vi "BDSCTRL_Write_Configuration_Settings_File.vi"(0 "configuration file path":path, 1 "BDSCTRL Connection Settings":T9={"Panel IP Address"="10.1.11.247", "Melvitron IP Address"="COM12", "EXA IP Address"="10.1.11.123", "MXG IP Address"="10.1.11.122"}, 2 "Test Setup Settings":T8={"IF Calibration File"=path "IFCalExample.csv", "Beam Lookup Table"=path "BeamLookupTableExample.csv", "Test Environment"=enum."Melvitron", "Panel Mode"=enum."CPRI", "Calibration Mode"=0, "Panel Type"=0, "Band"=0, "Tile"=0, "API Drop"=0} {"API Drop" items=["MAY", "JUNE"]; "Tile" items=["HP-C", "HP-B3"]; "Band" items=["AWS", "PCS-A", "PCS-G"]; "Panel Type" items=["Half", "Full", "Quarter"]; "Calibration Mode" items=["Manual", "SemiAuto", "Auto"]}, 3 "Panel Action Sequence":T6[](array[typedef]) items=["Panel Init", "RF Calibration", "Rotate Beam", "Set RF Frequency", "Initial Calibrations", "Channel Enable", "IF Calibration", "Sense Power", "Measure Temperature", "Set RF Power Level", "Run DMA", "Set RF Bandwidth", "Set CFR", "Set Beam"], 5 "error in \n(no error)":errorcluster, 6 "Channels Cluster":T7={"TX1"=TRUE, "TX2"=TRUE, "TX3"=FALSE, "TX4"=FALSE, "TXx3"=TRUE, "TXx4"=TRUE, "RX1"=FALSE, "RX2"=FALSE, "RX3"=FALSE, "RX4"=FALSE, "RXx3"=FALSE, "RXx4"=FALSE, "Tx"=TRUE, "Rx"=FALSE}, 7 "Set Beam Settings Cluster":T3, 8 "Beam Rotation":string[][](table)=[["1"], ["1"], ["1"], ["1"], ["1"], ["1"], ["2"], ["2"], ["2"], ["2"], ["2"], ["2"]], 9 "DMA Settings Cluster":T2, 10 "Target Devices Cluster":T5={"Target Devices"={"P1 Cluster"={"P1_D1"=TRUE, "P1_D2"=TRUE, "P1_D3"=TRUE, "P1_D4"=TRUE, "P1_D5"=TRUE, "P1_D6"=TRUE, "P1_D7"=TRUE, "P1_D8"=TRUE, "P1_D9"=TRUE, "P1_D10"=TRUE, "P1_D11"=TRUE, "P1_D12"=TRUE, "P1_D13"=TRUE, "P1_D14"=TRUE, "P1_D15"=TRUE, "P1_D16"=TRUE, "P1_D17"=TRUE, "P1_D18"=TRUE, "P1_D19"=TRUE, "P1_D20"=TRUE, "P1_D21"=TRUE, "P1_D22"=TRUE, "P1_D23"=TRUE, "P1_D24"=TRUE}, "P2 Cluster"={"P2_D1"=TRUE, "P2_D2"=TRUE, "P2_D3"=TRUE, "P2_D4"=TRUE, "P2_D5"=TRUE, "P2_D6"=TRUE, "P2_D7"=TRUE, "P2_D8"=TRUE, "P2_D9"=TRUE, "P2_D10"=TRUE, "P2_D11"=TRUE, "P2_D12"=TRUE, "P2_D13"=TRUE, "P2_D14"=TRUE, "P2_D15"=TRUE, "P2_D16"=TRUE, "P2_D17"=TRUE, "P2_D18"=TRUE, "P2_D19"=TRUE, "P2_D20"=TRUE, "P2_D21"=TRUE, "P2_D22"=TRUE, "P2_D23"=TRUE, "P2_D24"=TRUE}}, "Target String"="{1:24,1:24,[],[]}"}, 11 "MB-CFR Settings Cluster":T1, 12 "RF Parameters Settings Cluster":T4={"Tx RF \nFrequency"=2132.5, "RF Bandwidth \n(MHz)"=0, "Tx VGA"=[], "Rx VGA"=[]}) -> (19 "error out":errorcluster)   [LabVIEW 2016]
doc: "Illustrates how to create and write a configuration settings file.\n\nInstructions:\nEnter values in the controls on the front panel then click on the Run Arrow.\nTo read the file, run Read Configuration Settings File.vi located in the file\\config.llb."
uses:
  BDSCTRL_Controls/BDSCTRL_Panel_Action_List.ctl
  <vilib>/Utility/config.llb/Write Key (String).vi
  <vilib>/Utility/config.llb/Write Key (Path).vi
  <vilib>/Utility/config.llb/Write Key (I32).vi
  <vilib>/Utility/config.llb/Write Key (U32).vi
  <vilib>/Utility/config.llb/Write Key (Boolean).vi
  <vilib>/Utility/config.llb/Write Key (Double).vi
  <vilib>/Utility/config.llb/NI_LVConfig.lvlib
panel:
  in  "Instrument Mode Cluster":T10
  out "Array Indexing":string[](array[string])=["A", "B", "C", "D", "E", "F"]
  in  "Test Array":T11(array[cluster])=[{"Test Module"=0, "Select"=TRUE, "Configure\nParameters"=FALSE}, {"Test Module"=0, "Select"=FALSE, "Configure\nParameters"=FALSE}, {"Test Module"=0, "Select"=FALSE, "Configure\nParameters"=FALSE}, {"Test Module"=0, "Select"=FALSE, "Configure\nParameters"=FALSE}, {"Test Module"=0, "Select"=FALSE, "Configure\nParameters"=FALSE}, {"Test Module"=0, "Select"=FALSE, "Configure\nParameters"=FALSE}, {"Test Module"=0, "Select"=FALSE, "Configure\nParameters"=FALSE}, {"Test Module"=0, "Select"=FALSE, "Configure\nParameters"=FALSE}, {"Test Module"=0, "Select"=FALSE, "Configure\nParameters"=FALSE}, {"Test Module"=0, "Select"=FALSE, "Configure\nParameters"=FALSE}, {"Test Module"=0, "Select"=FALSE, "Configure\nParameters"=FALSE}, {"Test Module"=0, "Select"=FALSE, "Configure\nParameters"=FALSE}, {"Test Module"=0, "Select"=FALSE, "Configure\nParameters"=FALSE}, {"Test Module"=0, "Select"=FALSE, "Configure\nParameters"=FALSE}, {"Test Module"=0, "Select"=FALSE, "Configure\nParameters"=FALSE}, {"Test Module"=0, "Select"=FALSE, "Configure\nParameters"=FALSE}, {"Test Module"=0, "Select"=FALSE, "Configure\nParameters"=FALSE}, {"Test Module"=0, "Select"=FALSE, "Configure\nParameters"=FALSE}, {"Test Module"=0, "Select"=FALSE, "Configure\nParameters"=FALSE}, {"Test Module"=0, "Select"=FALSE, "Configure\nParameters"=FALSE}] {"Test Module" items=["::Select_a_module::", "Dynamic_Range", "EVM_FreqErr_OutputPower_GainFlatness", "RSSI"]}
  # "P2"
  # "P1"
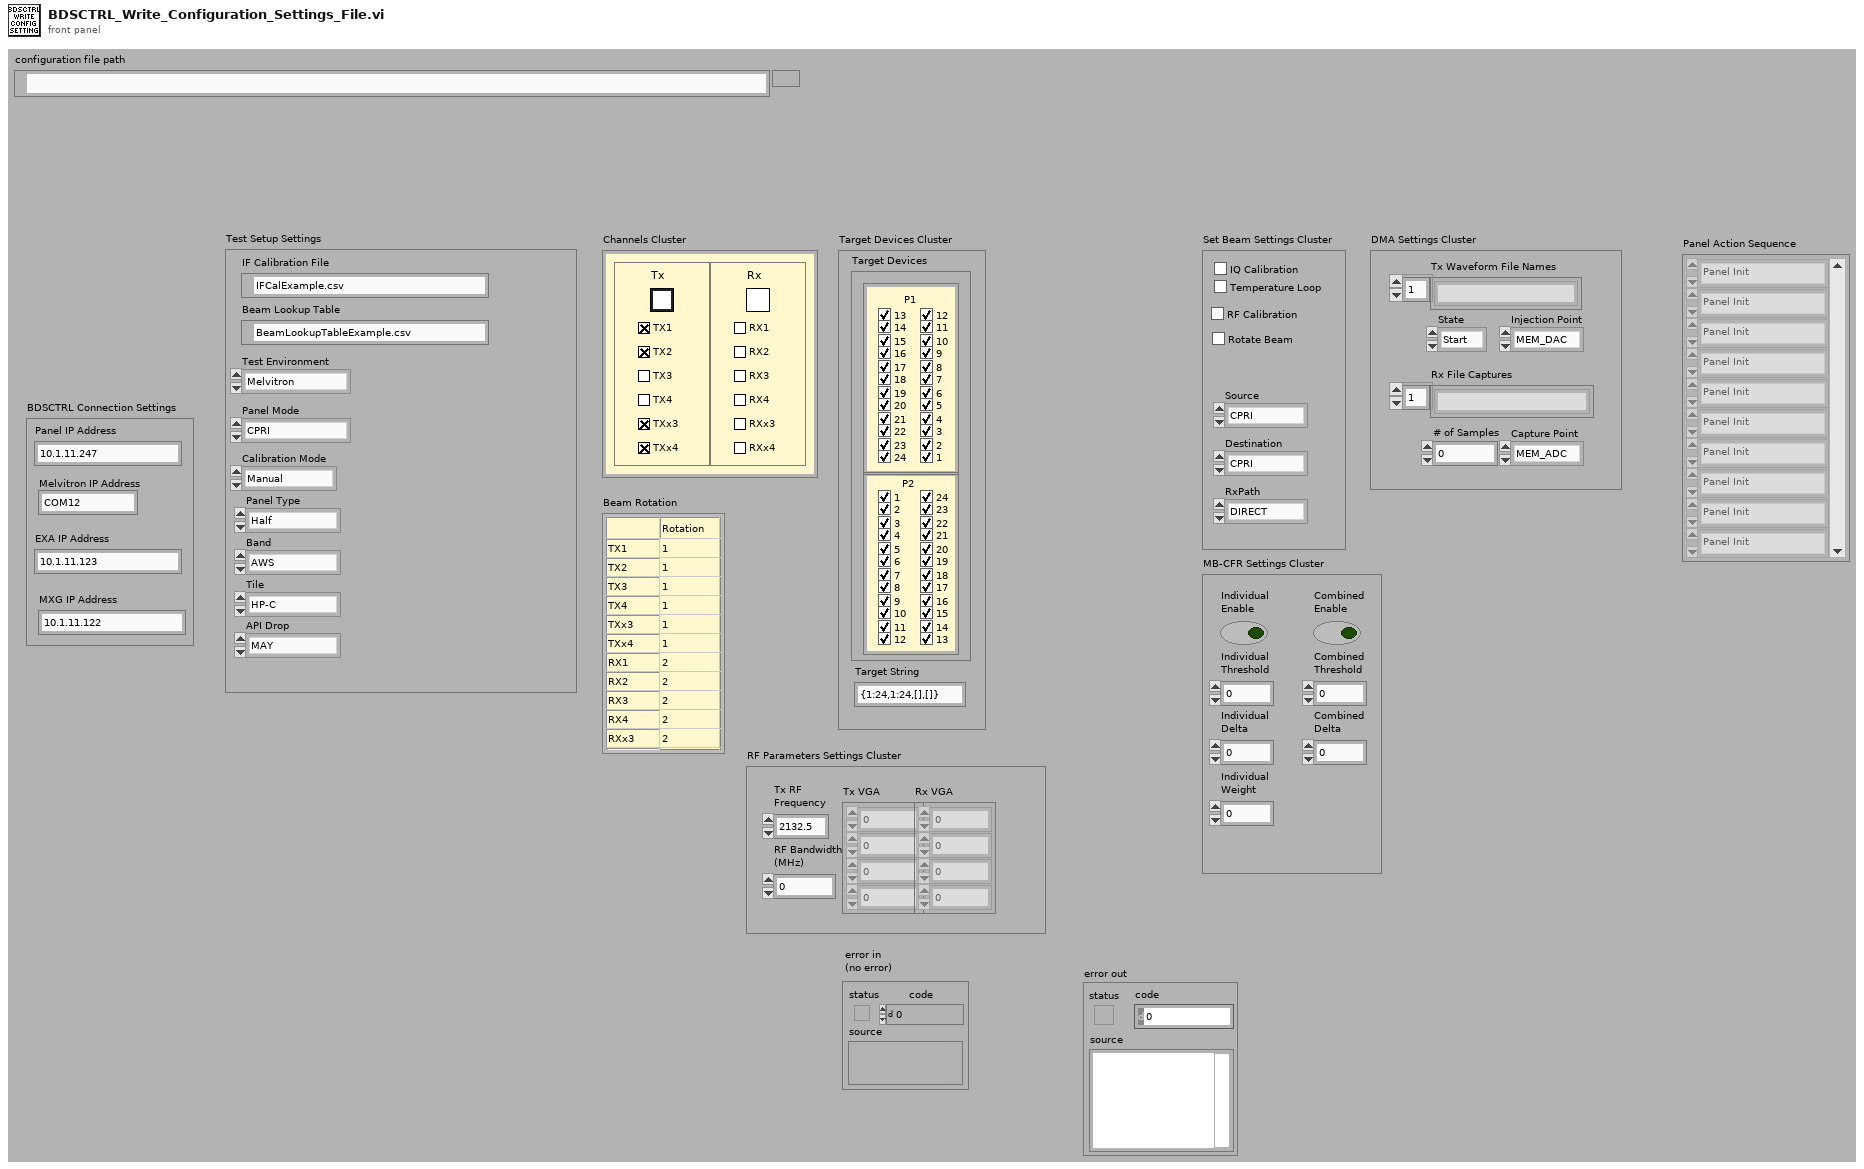
[diagram p1: front panel]
types:
  T1 = cluster{"Individual\nEnable":bool, "Individual\nThreshold":dbl, "Individual\nDelta":dbl, "Individual\nWeight":dbl, "Combined\nEnable":bool, "Combined\nThreshold":dbl, "Combined\nDelta":dbl}
  T2 = cluster{"Tx Waveform File Names":string[], "State":enum16{"Start", "Stop"}, "Injection Point":enum16{"MEM_DAC", "MEM_DUC"}, "Rx File Captures":string[], "# of Samples":i32, "Capture Point":enum16{"MEM_ADC", "MEM_DDC"}}
  T3 = cluster{"IQ Calibration":bool, "Temperature Loop":bool, "RF Calibration":bool, "Rotate Beam":bool, "Source":enum16{"CPRI", "CAL", "MEM_DAC", "MEM_DUC", "EXT"}, "Destination":enum16{"CPRI", "EXT", "MEM_ADC", "MEM_DDC"}, "RxPath":enum16{"DIRECT", "MIXER"}}
  T4 = cluster{"Tx RF \nFrequency":dbl, "RF Bandwidth \n(MHz)":i32, "Tx VGA":i32[], "Rx VGA":i32[]}
  T5 = cluster{"Target Devices":cluster{"P1 Cluster":cluster{"P1_D1":bool, "P1_D2":bool, "P1_D3":bool, "P1_D4":bool, "P1_D5":bool, "P1_D6":bool, "P1_D7":bool, "P1_D8":bool, "P1_D9":bool, "P1_D10":bool, "P1_D11":bool, "P1_D12":bool, "P1_D13":bool, "P1_D14":bool, "P1_D15":bool, "P1_D16":bool, "P1_D17":bool, "P1_D18":bool, "P1_D19":bool, "P1_D20":bool, "P1_D21":bool, "P1_D22":bool, "P1_D23":bool, "P1_D24":bool}, "P2 Cluster":cluster{"P2_D1":bool, "P2_D2":bool, "P2_D3":bool, "P2_D4":bool, "P2_D5":bool, "P2_D6":bool, "P2_D7":bool, "P2_D8":bool, "P2_D9":bool, "P2_D10":bool, "P2_D11":bool, "P2_D12":bool, "P2_D13":bool, "P2_D14":bool, "P2_D15":bool, "P2_D16":bool, "P2_D17":bool, "P2_D18":bool, "P2_D19":bool, "P2_D20":bool, "P2_D21":bool, "P2_D22":bool, "P2_D23":bool, "P2_D24":bool}}, "Target String":string}
  T6 = typedef "BDSCTRL_Panel_Action_List.ctl" = u16
  T7 = cluster{"TX1":bool, "TX2":bool, "TX3":bool, "TX4":bool, "TXx3":bool, "TXx4":bool, "RX1":bool, "RX2":bool, "RX3":bool, "RX4":bool, "RXx3":bool, "RXx4":bool, "Tx":bool, "Rx":bool}
  T8 = cluster{"IF Calibration File":path, "Beam Lookup Table":path, "Test Environment":enum16{"Melvitron", "Spider", "Marinotron"}, "Panel Mode":enum16{"CPRI", "UpDnCnv"}, "Calibration Mode":u16, "Panel Type":u16, "Band":u16, "Tile":u16, "API Drop":u16}
  T9 = cluster{"Panel IP Address":string, "Melvitron IP Address":string, "EXA IP Address":string, "MXG IP Address":string}
  T10 = cluster{"MXA Connection":cluster{"MXA":refnum<visa-resource-name>, "Entry Mode":enum16{"VISA", "IP Address"}}, "MXG1 Connection":cluster{"MXG 1":refnum<visa-resource-name>, "Entry Mode":enum16{"VISA", "IP Address"}}, "MXG2 Connection":cluster{"MXG 2":refnum<visa-resource-name>, "Entry Mode":enum16{"VISA", "IP Address"}}, "MXG3 Connection":cluster{"MXG 3":refnum<visa-resource-name>, "Entry Mode":enum16{"VISA", "IP Address"}}, "ENA Connection":cluster{"ENA":refnum<visa-resource-name>, "Entry Mode":enum16{"VISA", "IP Address"}}}
  T11 = cluster{"Test Module":u16, "Select":bool, "Configure\nParameters":bool}[]
  T12 = cluster{"MXA":refnum<visa-resource-name>, "Entry Mode":enum16{"VISA", "IP Address"}}
  T13 = cluster{"MXG 1":refnum<visa-resource-name>, "Entry Mode":enum16{"VISA", "IP Address"}}
  T14 = cluster{"MXG 2":refnum<visa-resource-name>, "Entry Mode":enum16{"VISA", "IP Address"}}
  T15 = cluster{"MXG 3":refnum<visa-resource-name>, "Entry Mode":enum16{"VISA", "IP Address"}}
  T16 = cluster{"ENA":refnum<visa-resource-name>, "Entry Mode":enum16{"VISA", "IP Address"}}
  T17 = typedef "NI_LVConfig.lvlib/Config Data RefNum.ctl" = refnum<k1>
  T18 = cluster{"P1 Cluster":cluster{"P1_D1":bool, "P1_D2":bool, "P1_D3":bool, "P1_D4":bool, "P1_D5":bool, "P1_D6":bool, "P1_D7":bool, "P1_D8":bool, "P1_D9":bool, "P1_D10":bool, "P1_D11":bool, "P1_D12":bool, "P1_D13":bool, "P1_D14":bool, "P1_D15":bool, "P1_D16":bool, "P1_D17":bool, "P1_D18":bool, "P1_D19":bool, "P1_D20":bool, "P1_D21":bool, "P1_D22":bool, "P1_D23":bool, "P1_D24":bool}, "P2 Cluster":cluster{"P2_D1":bool, "P2_D2":bool, "P2_D3":bool, "P2_D4":bool, "P2_D5":bool, "P2_D6":bool, "P2_D7":bool, "P2_D8":bool, "P2_D9":bool, "P2_D10":bool, "P2_D11":bool, "P2_D12":bool, "P2_D13":bool, "P2_D14":bool, "P2_D15":bool, "P2_D16":bool, "P2_D17":bool, "P2_D18":bool, "P2_D19":bool, "P2_D20":bool, "P2_D21":bool, "P2_D22":bool, "P2_D23":bool, "P2_D24":bool}}
  T19 = cluster{"P2_D1":bool, "P2_D2":bool, "P2_D3":bool, "P2_D4":bool, "P2_D5":bool, "P2_D6":bool, "P2_D7":bool, "P2_D8":bool, "P2_D9":bool, "P2_D10":bool, "P2_D11":bool, "P2_D12":bool, "P2_D13":bool, "P2_D14":bool, "P2_D15":bool, "P2_D16":bool, "P2_D17":bool, "P2_D18":bool, "P2_D19":bool, "P2_D20":bool, "P2_D21":bool, "P2_D22":bool, "P2_D23":bool, "P2_D24":bool}[]
  T20 = cluster{"P2_D1":bool, "P2_D2":bool, "P2_D3":bool, "P2_D4":bool, "P2_D5":bool, "P2_D6":bool, "P2_D7":bool, "P2_D8":bool, "P2_D9":bool, "P2_D10":bool, "P2_D11":bool, "P2_D12":bool, "P2_D13":bool, "P2_D14":bool, "P2_D15":bool, "P2_D16":bool, "P2_D17":bool, "P2_D18":bool, "P2_D19":bool, "P2_D20":bool, "P2_D21":bool, "P2_D22":bool, "P2_D23":bool, "P2_D24":bool}
  T21 = enum16{"CPRI", "CAL", "MEM_DAC", "MEM_DUC", "EXT"}
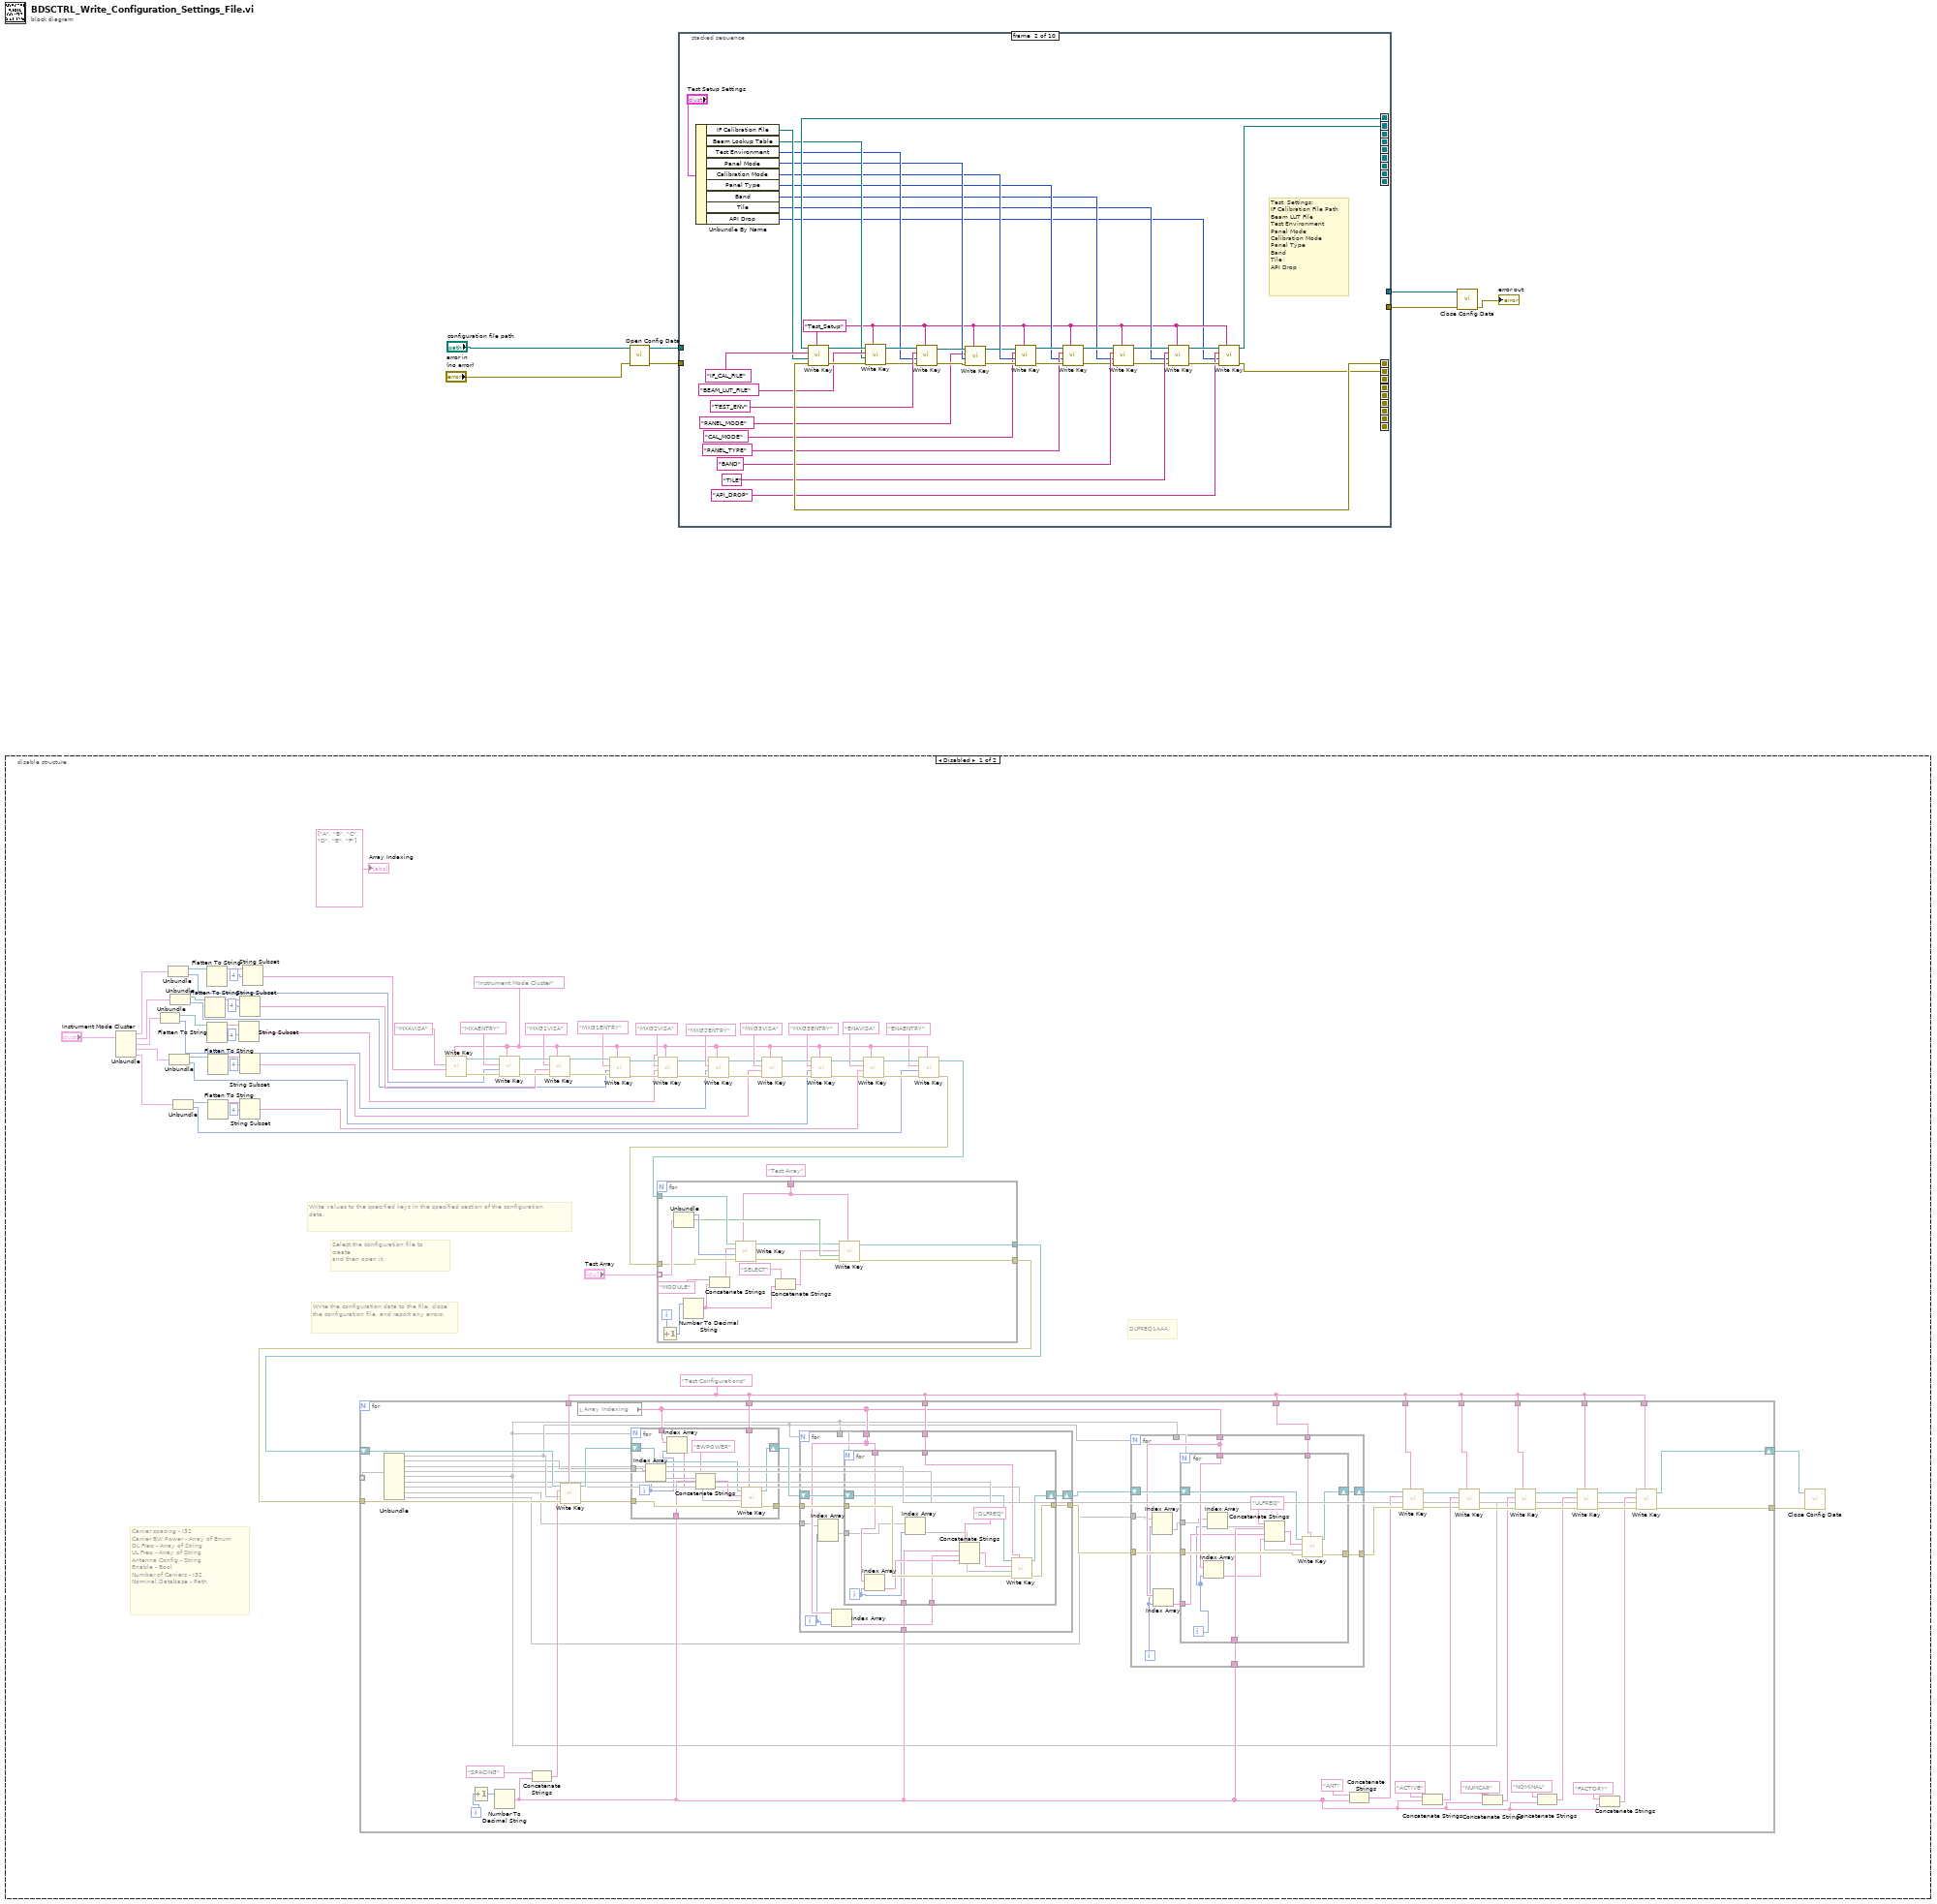
[diagram p0: block diagram]
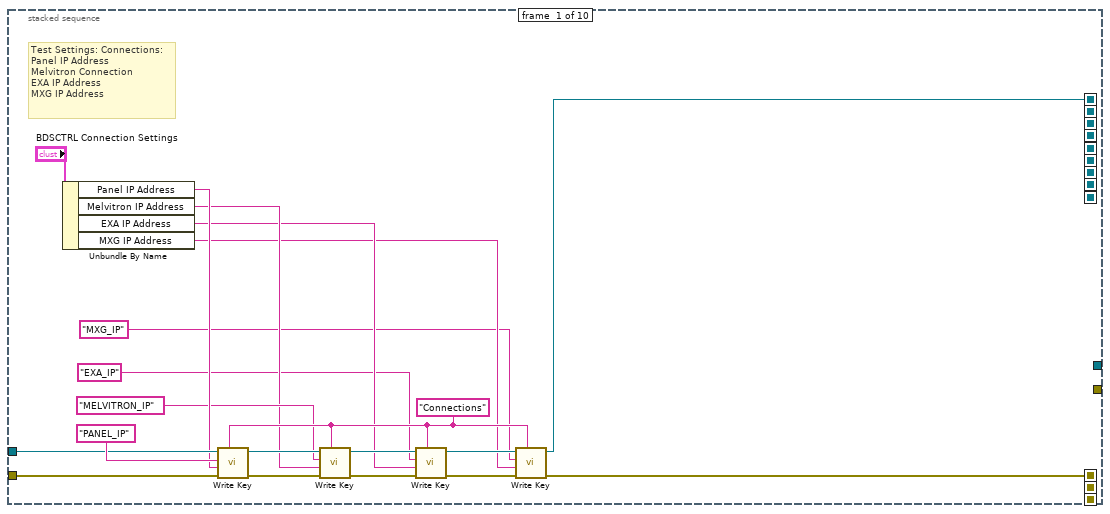
[diagram p3: hidden frame]
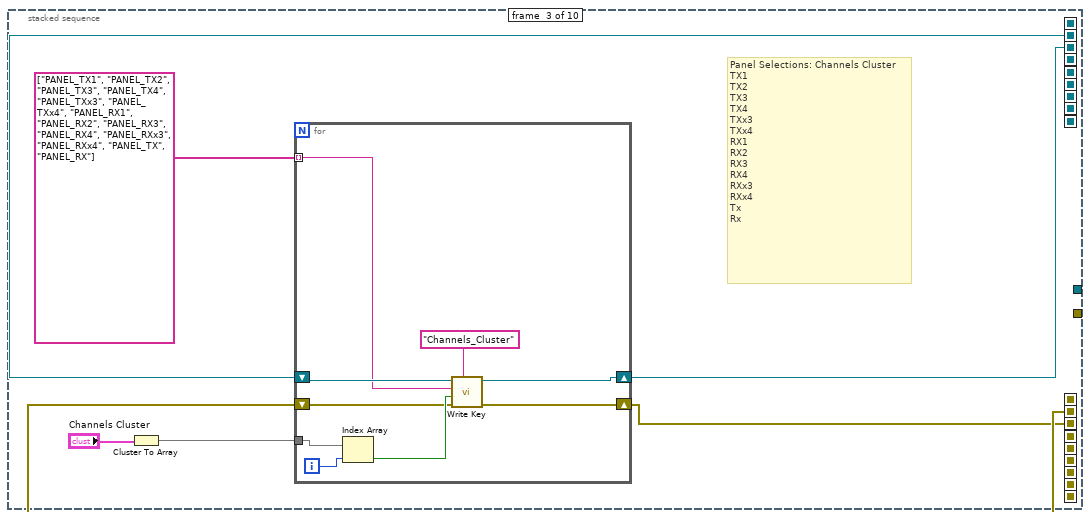
[diagram p4: hidden frame]
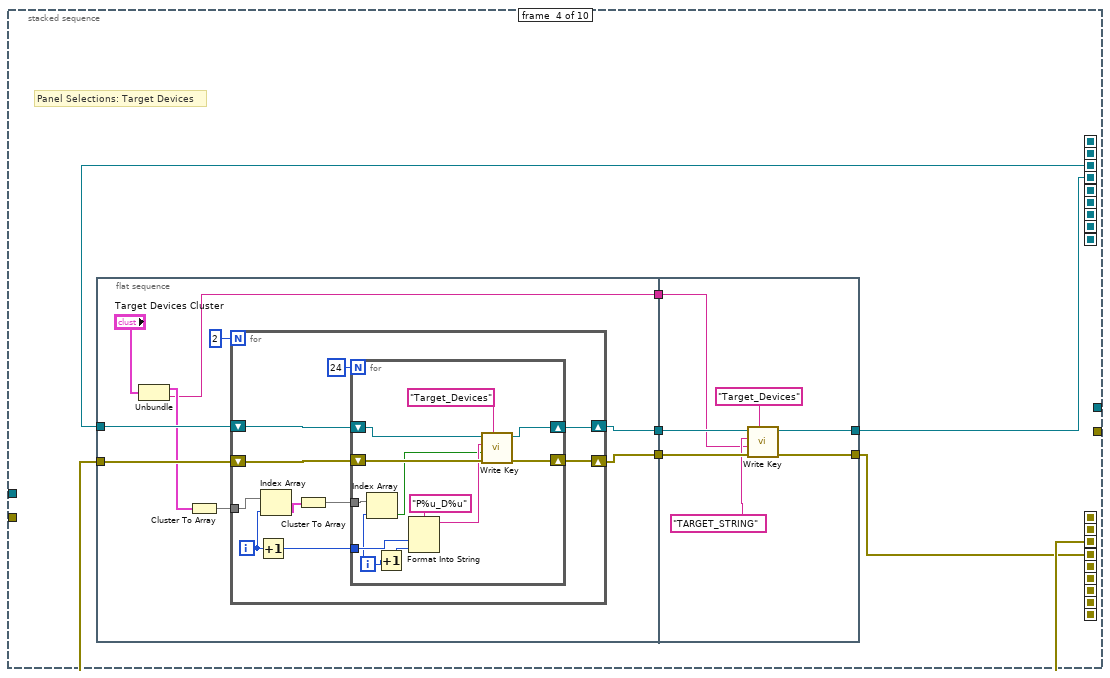
[diagram p5: hidden frame]
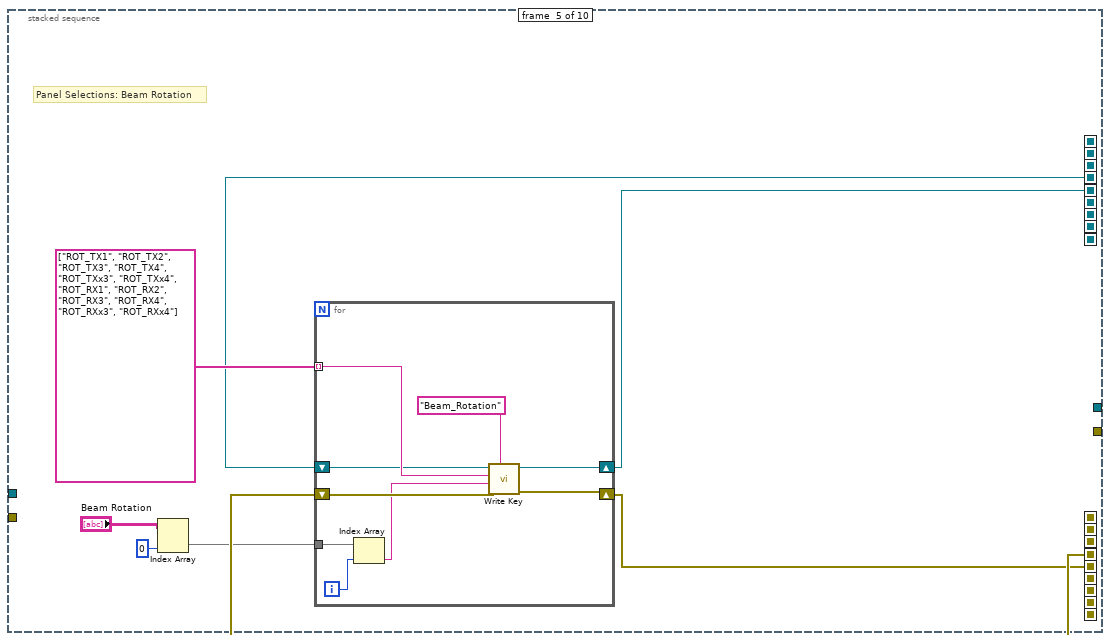
[diagram p6: hidden frame]
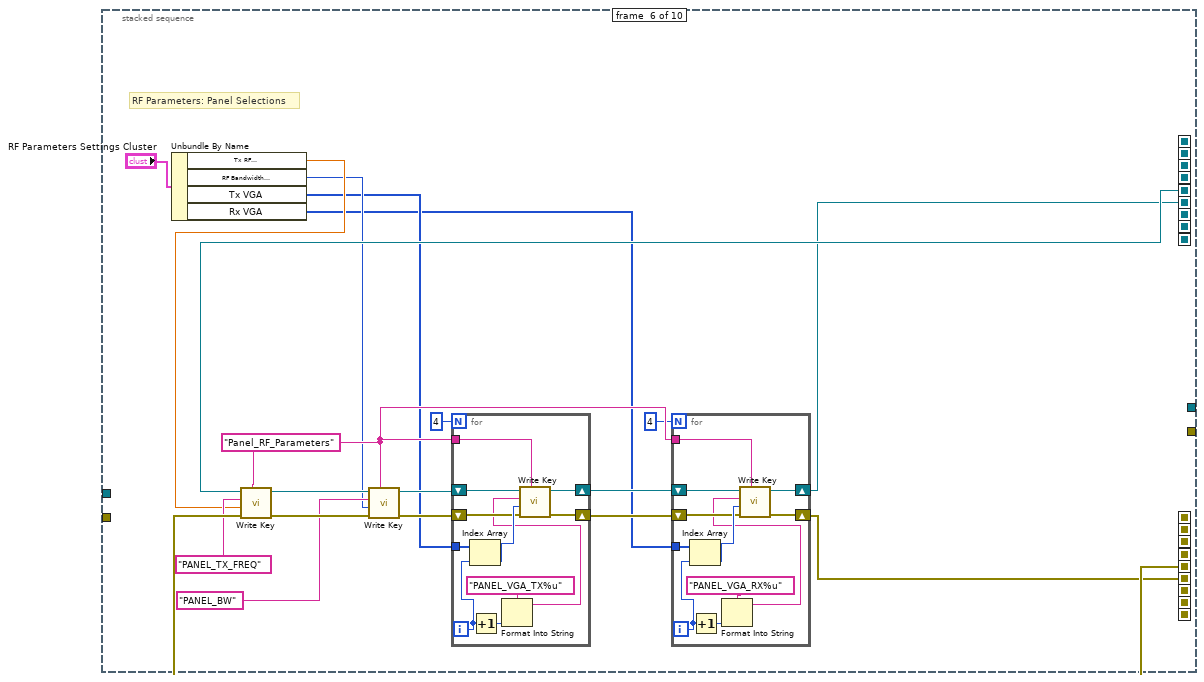
[diagram p7: hidden frame]
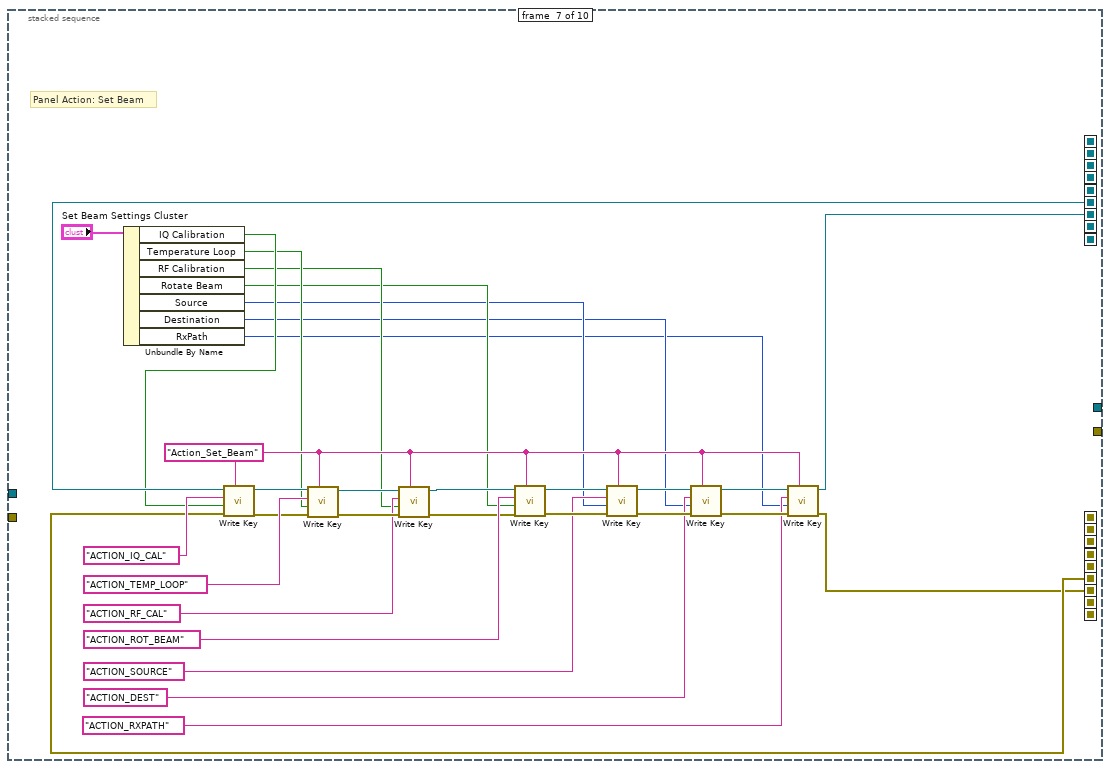
[diagram p8: hidden frame]
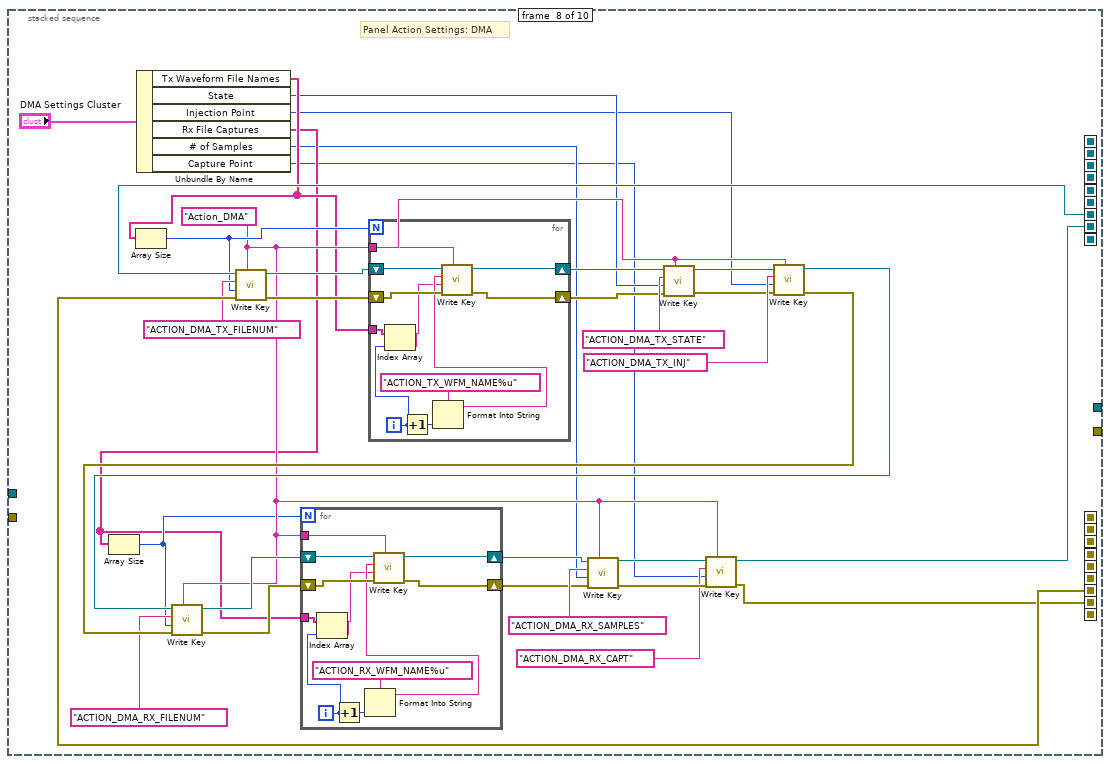
[diagram p9: hidden frame]
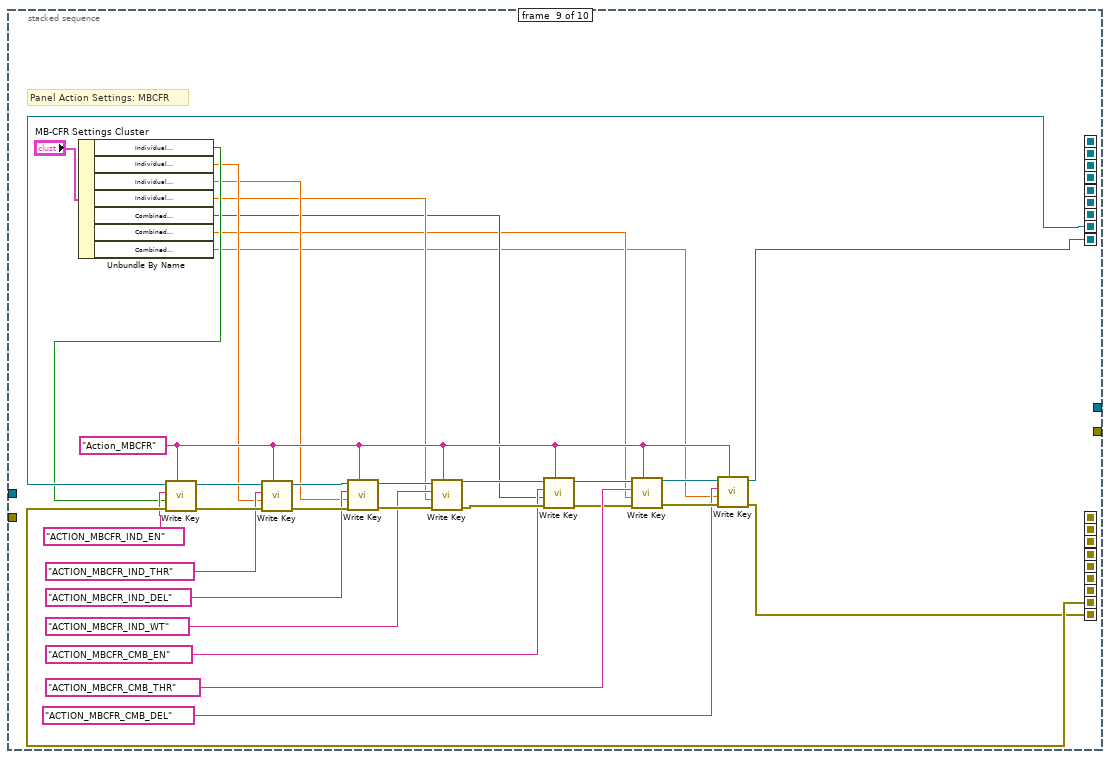
[diagram p10: hidden frame]
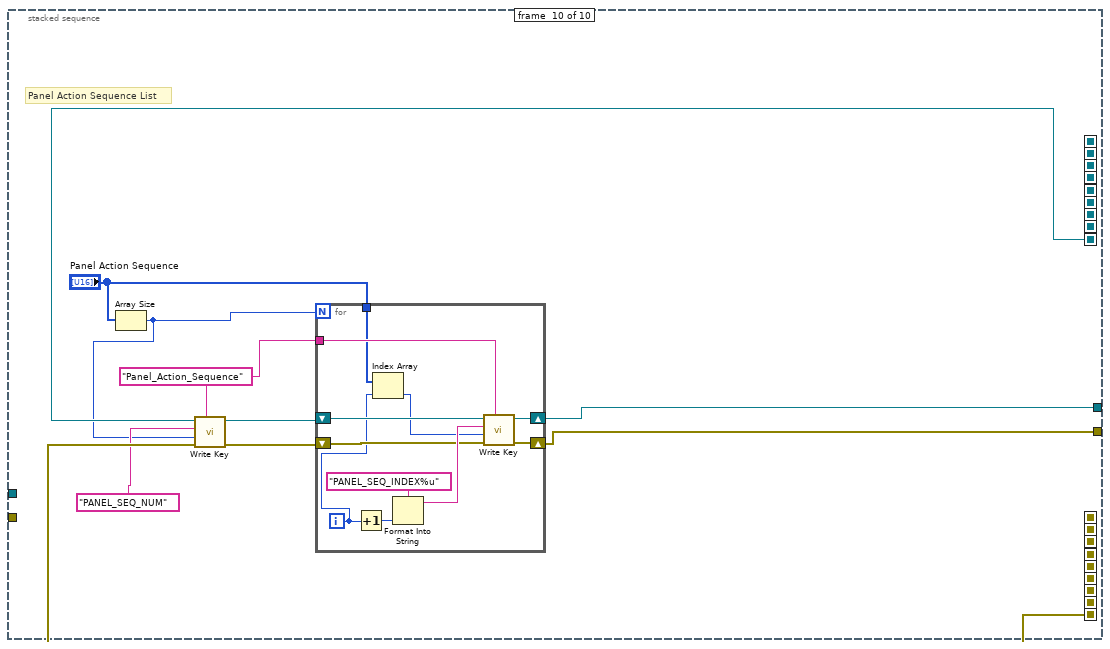
[diagram p11: hidden frame]
diagram:
  n1 = disable-structure shown="Disabled" {
    frame Disabled {
      w12 = "Instrument Mode Cluster" ("section")
      w72 = "Test Configurations" ("section")
      # "DLFREQ1AAA"
      # "Carrier spacing - I32\nCarrier BW Power - Array of Enum\nDL Freq - Array of String\nUL Freq - Array of String\nAntenna Config - String\nEnable - Bool\nNumber of Carriers - I32\nNominal Database - Path"
      # "Write the configuration data to the file, close the configuration file, and report any errors."
      # "Write values to the specified keys in the specified section of the configuration data."
      # "Select the configuration file to create\nand then open it."
      n2 = Unbundle("Instrument Mode Cluster") -> ("MXA Connection"=w70:T12, "MXG1 Connection"=w69:T13, "MXG2 Connection"=w68:T14, "MXG3 Connection"=w67:T15, "ENA Connection"=w66:T16)
      n3 = Unbundle(w68) -> ("MXG 2"=w55:refnum<visa-resource-name>, "Entry Mode"=w26:enum16{"VISA", "IP Address"})
      n4 = Unbundle(w70) -> ("MXA"=w61:refnum<visa-resource-name>, "Entry Mode"=w43:enum16{"VISA", "IP Address"})
      n5 = Unbundle(w67) -> ("MXG 3"=w53:refnum<visa-resource-name>, "Entry Mode"=w20:enum16{"VISA", "IP Address"})
      n6 = Unbundle(w69) -> ("MXG 1"=w58:refnum<visa-resource-name>, "Entry Mode"=w31:enum16{"VISA", "IP Address"})
      n7 = Unbundle(w66) -> ("ENA"=w51:refnum<visa-resource-name>, "Entry Mode"=w10:enum16{"VISA", "IP Address"})
      n8 = Flatten To String(anything=w58) -> (data string=w60:string)  [unwired: 3 in, 2 out]
      n9 = Flatten To String(anything=w61) -> (data string=w62:string)  [unwired: 3 in, 2 out]
      n10 = Flatten To String(anything=w55) -> (data string=w56:string)  [unwired: 3 in, 2 out]
      n11 = Flatten To String(anything=w53) -> (data string=w52:string)  [unwired: 3 in, 2 out]
      n12 = Flatten To String(anything=w51) -> (data string=w49:string)  [unwired: 3 in, 2 out]
      n13 = String Subset(string=w56, offset (0)=4) -> (substring=w32:string)  [unwired: 1 in]
      n14 = String Subset(string=w52, offset (0)=4) -> (substring=w23:string)  [unwired: 1 in]
      n15 = String Subset(string=w60, offset (0)=4) -> (substring=w39:string)  [unwired: 1 in]
      n16 = String Subset(string=w49, offset (0)=4) -> (substring=w17:string)  [unwired: 1 in]
      n17 = String Subset(string=w62, offset (0)=4) -> (substring=w47:string)  [unwired: 1 in]
      n18 = call-poly <vilib>:"Write Key.vi"("section"=w12, "value"=w47, "key"="MXAVISA") -> ("error out"=w45:errorcluster, "refnum out"=w46:T17, "error in (no error)"=w64:errorcluster, "refnum"=w65:T17)  [unwired: 4 in, 1 out]
      n19 = call-poly <vilib>:"Write Key.vi"("section"=w12, "error in (no error)"=w45, "value"=w43, "key"="MXAENTRY", "refnum"=w46) -> ("error out"=w41:errorcluster, "refnum out"=w42:T17)  [unwired: 4 in, 1 out]
      n20 = call-poly <vilib>:"Write Key.vi"("section"=w12, "error in (no error)"=w41, "value"=w39, "key"="MXG1VISA", "refnum"=w42) -> ("error out"=w38:errorcluster, "refnum out"=w37:T17)  [unwired: 4 in, 1 out]
      n21 = call-poly <vilib>:"Write Key.vi"("section"=w12, "error in (no error)"=w38, "value"=w31, "key"="MXG1ENTRY", "refnum"=w37) -> ("error out"=w34:errorcluster, "refnum out"=w35:T17)  [unwired: 4 in, 1 out]
      n22 = call-poly <vilib>:"Write Key.vi"("section"=w12, "error in (no error)"=w34, "value"=w32, "key"="MXG2VISA", "refnum"=w35) -> ("error out"=w30:errorcluster, "refnum out"=w27:T17)  [unwired: 4 in, 1 out]
      n23 = call-poly <vilib>:"Write Key.vi"("section"=w12, "error in (no error)"=w30, "value"=w26, "key"="MXG2ENTRY", "refnum"=w27) -> ("error out"=w29:errorcluster, "refnum out"=w24:T17)  [unwired: 4 in, 1 out]
      n24 = call-poly <vilib>:"Write Key.vi"("section"=w12, "error in (no error)"=w29, "value"=w23, "key"="MXG3VISA", "refnum"=w24) -> ("error out"=w22:errorcluster, "refnum out"=w21:T17)  [unwired: 4 in, 1 out]
      n25 = call-poly <vilib>:"Write Key.vi"("section"=w12, "error in (no error)"=w22, "value"=w20, "key"="MXG3ENTRY", "refnum"=w21) -> ("error out"=w16:errorcluster, "refnum out"=w15:T17)  [unwired: 4 in, 1 out]
      n26 = call-poly <vilib>:"Write Key.vi"("section"=w12, "error in (no error)"=w16, "value"=w17, "key"="ENAVISA", "refnum"=w15) -> ("error out"=w14:errorcluster, "refnum out"=w13:T17)  [unwired: 4 in, 1 out]
      n27 = call-poly <vilib>:"Write Key.vi"("section"=w12, "error in (no error)"=w14, "value"=w10, "key"="ENAENTRY", "refnum"=w13) -> ("error out"=w8:errorcluster, "refnum out"=w9:T17)  [unwired: 4 in, 1 out]
      n28 = for {
        tunnel: "Test Array" ("section") -> [w205]
        tunnel: [w202] -> w75
        tunnel: [w203] -> w77
        tunnel: "Test Array" -> [w215] mode=indexing
        tunnel: w8 -> [w214]
        tunnel: w9 -> [w211]
        i -> [w218]
        n29 = Increment(x=w218) -> (x+1=w216:i32)
        n30 = Unbundle(w215) -> ("Test Module"=w213:u16, "Select"=w208:bool)  [unwired: 1 out]
        n31 = Number To Decimal String(number=w216) -> (decimal integer string=w209:string)  [unwired: 1 in]
        n32 = Concatenate Strings("MODULE", w209) -> (w212:string)
        n33 = call-poly <vilib>:"Write Key.vi"("section"=w205, "error in (no error)"=w214, "value"=w213, "key"=w212, "refnum"=w211) -> ("error out"=w204:errorcluster, "refnum out"=w207:T17)  [unwired: 4 in, 1 out]
        n34 = Concatenate Strings("SELECT", w209) -> (w206:string)
        n35 = call-poly <vilib>:"Write Key.vi"("section"=w205, "error in (no error)"=w204, "value"=w208, "key"=w206, "refnum"=w207) -> ("error out"=w203:errorcluster, "refnum out"=w202:T17)  [unwired: 4 in, 1 out]
      }
      n36 = for {
        tunnel: [w136] -> w78 mode=indexing
        tunnel: w77 -> [w133]
        tunnel: w72 -> [w132]
        tunnel: w72 -> [w127]
        tunnel: w72 -> [w125]
        tunnel: w72 -> [w122]
        tunnel: w72 -> [w118]
        tunnel: w72 -> [w111]
        tunnel: w72 -> [w108]
        shift-right: [w91] -> w73
        shift-left: w75 -> [w105]
        tunnel: [w90] -> w74
        tunnel: w72 -> [w101]
        tunnel: w72 -> [w99]
        i -> [w134]
        n37 = Unbundle(w136) -> (w87, w130, w86, w85, w84, w83, w82, w89, w88)
        n38 = Increment(x=w134) -> (x+1=w135:i32)
        n39 = Number To Decimal String(number=w135) -> (decimal integer string=w94:string)  [unwired: 1 in]
        n40 = Concatenate Strings("SPACING", w94) -> (w121:string)
        n41 = call-poly <vilib>:"Write Key.vi"("section"=w132, "error in (no error)"=w133, "value"=w87, "key"=w121, "refnum"=w105) -> ("error out"=w128:errorcluster, "refnum out"=w129:T17)  [unwired: 4 in, 1 out]
        n42 = local read "Array Indexing"() -> (w124:string[])
        n43 = for {
          N: w84 -> [_]
          tunnel: w130 -> [w201]
          shift-right: [w195] -> w104
          shift-left: w129 -> [w196]
          tunnel: w128 -> [w200]
          tunnel: w124 -> [w191]
          tunnel: w94 -> [w199]
          tunnel: w127 -> [w194]
          tunnel: [w192] -> w126
          i -> [w190]
          n44 = Index Array(array=w201, index=w190) -> (element=w193)
          n45 = Index Array(array=w191, index=w190) -> (element=w189:string)
          n46 = Concatenate Strings("BWPOWER", w199, w189) -> (w197:string)
          n47 = call-poly <vilib>:"Write Key.vi"("section"=w194, "error in (no error)"=w200, "value"=w193, "key"=w197, "refnum"=w196) -> ("error out"=w192:errorcluster, "refnum out"=w195:T17)  [unwired: 4 in, 1 out]
        }
        n48 = for {
          N: w87 -> [_]
          tunnel: w126 -> [w174]
          tunnel: w89 -> [w166]
          tunnel: w125 -> [w173]
          tunnel: w124 -> [w168]
          tunnel: [w171] -> w123
          tunnel: w94 -> [w170]
          shift-right: [w172] -> w103
          shift-left: w104 -> [w169]
          tunnel: w84 -> [w165]
          i -> [w164]
          n49 = Index Array(array=w166, index (row)=w164) -> (element=w163)  [unwired: 1 in]
          n50 = Index Array(array=w168, index=w164) -> (element=w167:string)
          n51 = for {
            N: w165 -> [_]
            tunnel: w174 -> [w188]
            tunnel: w173 -> [w187]
            tunnel: w168 -> [w182]
            tunnel: [w185] -> w171
            tunnel: w170 -> [w184]
            shift-right: [w186] -> w172
            shift-left: w169 -> [w183]
            tunnel: w167 -> [w178]
            tunnel: w163 -> [w177]
            i -> [w176]
            n52 = Index Array(array=w182, index=w176) -> (element=w179:string)
            n53 = Index Array(array=w177, index=w176) -> (element=w175)
            n54 = Concatenate Strings("DLFREQ", w184, w178, w179) -> (w180:string)
            n55 = call-poly <vilib>:"Write Key.vi"("section"=w187, "error in (no error)"=w188, "value"=w175, "key"=w180, "refnum"=w183) -> ("error out"=w185:errorcluster, "refnum out"=w186:T17)  [unwired: 4 in, 1 out]
          }
        }
        n56 = for {
          N: w87 -> [_]
          tunnel: w124 -> [w142]
          tunnel: w123 -> [w148]
          tunnel: w122 -> [w147]
          tunnel: w88 -> [w140]
          tunnel: [w146] -> w120
          tunnel: w94 -> [w144]
          shift-right: [w145] -> w119
          shift-left: w103 -> [w143]
          tunnel: w84 -> [w137]
          i -> [w139]
          n57 = Index Array(array=w140, index (row)=w139) -> (element=w138)  [unwired: 1 in]
          n58 = Index Array(array=w142, index=w139) -> (element=w141:string)
          n59 = for {
            N: w137 -> [_]
            tunnel: w142 -> [w156]
            tunnel: w148 -> [w162]
            tunnel: w147 -> [w161]
            tunnel: [w160] -> w146
            tunnel: w144 -> [w158]
            shift-right: [w159] -> w145
            shift-left: w143 -> [w157]
            tunnel: w141 -> [w153]
            tunnel: w138 -> [w151]
            i -> [w150]
            n60 = Index Array(array=w156, index=w150) -> (element=w152:string)
            n61 = Index Array(array=w151, index=w150) -> (element=w149)
            n62 = Concatenate Strings("ULFREQ", w158, w153, w152) -> (w154:string)
            n63 = call-poly <vilib>:"Write Key.vi"("section"=w161, "error in (no error)"=w162, "value"=w149, "key"=w154, "refnum"=w157) -> ("error out"=w160:errorcluster, "refnum out"=w159:T17)  [unwired: 4 in, 1 out]
          }
        }
        n64 = Concatenate Strings("ANT", w94) -> (w116:string)
        n65 = call-poly <vilib>:"Write Key.vi"("section"=w118, "error in (no error)"=w120, "value"=w86, "key"=w116, "refnum"=w119) -> ("error out"=w112:errorcluster, "refnum out"=w113:T17)  [unwired: 4 in, 1 out]
        n66 = Concatenate Strings("ACTIVE", w94) -> (w114:string)
        n67 = call-poly <vilib>:"Write Key.vi"("section"=w111, "error in (no error)"=w112, "value"=w85, "key"=w114, "refnum"=w113) -> ("error out"=w110:errorcluster, "refnum out"=w109:T17)  [unwired: 4 in, 1 out]
        n68 = Concatenate Strings("NUMCAR", w94) -> (w106:string)
        n69 = call-poly <vilib>:"Write Key.vi"("section"=w108, "error in (no error)"=w110, "value"=w84, "key"=w106, "refnum"=w109) -> ("error out"=w102:errorcluster, "refnum out"=w96:T17)  [unwired: 4 in, 1 out]
        n70 = Concatenate Strings("NOMINAL", w94) -> (w97:string)
        n71 = call-poly <vilib>:"Write Key.vi"("section"=w101, "error in (no error)"=w102, "value"=w83, "key"=w97, "refnum"=w96) -> ("error out"=w100:errorcluster, "refnum out"=w92:T17)  [unwired: 4 in, 1 out]
        n72 = Concatenate Strings("FACTORY", w94) -> (w93:string)
        n73 = call-poly <vilib>:"Write Key.vi"("section"=w99, "error in (no error)"=w100, "value"=w82, "key"=w93, "refnum"=w92) -> ("error out"=w90:errorcluster, "refnum out"=w91:T17)  [unwired: 4 in, 1 out]
      }
      n74 = call <vilib>:"Close Config Data.vi"("error in (no error)"=w74, "refnum"=w73) -> ("error out"=w81:errorcluster)  [unwired: 1 in, 8 out]
      "Array Indexing" <- string[] ["A", "B", "C", "D", "E", "F"]
    }
    frame Enabled {
    }
  }
  n75 = call <vilib>:"Open Config Data.vi"("error in (no error)"="error in \n(no error)", "configuration file path"="configuration file path") -> ("error out"=w4:errorcluster, "refnum"=w5:T17)  [unwired: 1 in, 7 out]
  n76 = stacked-sequence {
    seq-local: [w220 _ _ _ _ _ _ _ _ _] -> [_ w276 _ _ _ _ _ _ _ _]
    seq-local: [w219 _ _ _ _ _ _ _ _ _] -> [_ w277 _ _ _ _ _ _ _ _]
    seq-local: [_ w240 _ _ _ _ _ _ _ _] -> [_ _ w281 _ _ _ _ _ _ _]
    seq-local: [_ w239 _ _ _ _ _ _ _ _] -> [_ _ w282 _ _ _ _ _ _ _]
    seq-local: [_ _ w279 _ _ _ _ _ _ _] -> [_ _ _ w301 _ _ _ _ _ _]
    seq-local: [_ _ w280 _ _ _ _ _ _ _] -> [_ _ _ w300 _ _ _ _ _ _]
    seq-local: [_ _ _ w297 _ _ _ _ _ _] -> [_ _ _ _ w345 _ _ _ _ _]
    seq-local: [_ _ _ w296 _ _ _ _ _ _] -> [_ _ _ _ w346 _ _ _ _ _]
    seq-local: [_ _ _ _ w341 _ _ _ _ _] -> [_ _ _ _ _ w374 _ _ _ _]
    seq-local: [_ _ _ _ w340 _ _ _ _ _] -> [_ _ _ _ _ w376 _ _ _ _]
    seq-local: [_ _ _ _ _ w363 _ _ _ _] -> [_ _ _ _ _ _ w430 _ _ _]
    seq-local: [_ _ _ _ _ w362 _ _ _ _] -> [_ _ _ _ _ _ w428 _ _ _]
    seq-local: [_ _ _ _ _ _ w407 _ _ _] -> [_ _ _ _ _ _ _ w463 _ _]
    seq-local: [_ _ _ _ _ _ w408 _ _ _] -> [_ _ _ _ _ _ _ w464 _ _]
    seq-local: [_ _ _ _ _ _ _ w440 _ _] -> [_ _ _ _ _ _ _ _ w517 _]
    seq-local: [_ _ _ _ _ _ _ w439 _ _] -> [_ _ _ _ _ _ _ _ w518 _]
    seq-local: [_ _ _ _ _ _ _ _ w496 _] -> [_ _ _ _ _ _ _ _ _ w528]
    seq-local: [_ _ _ _ _ _ _ _ w495 _] -> [_ _ _ _ _ _ _ _ _ w527]
    tunnel: w5 -> [w231 _ _ _ _ _ _ _ _ _]
    tunnel: w4 -> [w230 _ _ _ _ _ _ _ _ _]
    tunnel: [_ _ _ _ _ _ _ _ _ w521] -> w2
    tunnel: [_ _ _ _ _ _ _ _ _ w520] -> w1
    frame #0 {
      w229 = "Connections" ("section")
      # "Test Settings: Connections:\nPanel IP Address\nMelvitron Connection\nEXA IP Address\nMXG IP Address"
      n77 = Unbundle By Name("BDSCTRL Connection Settings") -> ("Panel IP Address"=w227:string, "Melvitron IP Address"=w225:string, "EXA IP Address"=w224:string, "MXG IP Address"=w222:string)
      n78 = call-poly <vilib>:"Write Key.vi"("section"=w229, "error in (no error)"=w230, "value"=w227, "key"="PANEL_IP", "refnum"=w231) -> ("error out"=w235:errorcluster, "refnum out"=w238:T17)  [unwired: 4 in, 1 out]
      n79 = call-poly <vilib>:"Write Key.vi"("section"=w229, "error in (no error)"=w235, "value"=w225, "key"="MELVITRON_IP", "refnum"=w238) -> ("error out"=w234:errorcluster, "refnum out"=w237:T17)  [unwired: 4 in, 1 out]
      n80 = call-poly <vilib>:"Write Key.vi"("section"=w229, "error in (no error)"=w234, "value"=w224, "key"="EXA_IP", "refnum"=w237) -> ("error out"=w233:errorcluster, "refnum out"=w236:T17)  [unwired: 1 in, 4 out]
      n81 = call-poly <vilib>:"Write Key.vi"("section"=w229, "error in (no error)"=w233, "value"=w222, "key"="MXG_IP", "refnum"=w236) -> ("error out"=w219:errorcluster, "refnum out"=w220:T17)  [unwired: 1 in, 4 out]
    }
    frame #1 {
      w243 = "Test_Setup" ("section")
      # "Test  Settings:\nIF Calibration File Path\nBeam LUT File\nTest Environment\nPanel Mode\nCalibration Mode\nPanel Type\nBand\nTile\nAPI Drop"
      n82 = Unbundle By Name("Test Setup Settings") -> ("IF Calibration File"=w273:path, "Beam Lookup Table"=w270:path, "Test Environment"=w266:enum16{"Melvitron", "Spider", "Marinotron"}, "Panel Mode"=w263:enum16{"CPRI", "UpDnCnv"}, "Calibration Mode"=w261:u16, "Panel Type"=w254:u16, "Band"=w251:u16, "Tile"=w246:u16, "API Drop"=w241:u16)
      n83 = call-poly <vilib>:"Write Key.vi"("section"=w243, "error in (no error)"=w277, "value"=w273, "key"="IF_CAL_FILE", "refnum"=w276) -> ("error out"=w272:errorcluster, "refnum out"=w274:T17)  [unwired: 4 in, 1 out]
      n84 = call-poly <vilib>:"Write Key.vi"("section"=w243, "error in (no error)"=w272, "value"=w270, "key"="BEAM_LUT_FILE", "refnum"=w274) -> ("error out"=w268:errorcluster, "refnum out"=w267:T17)  [unwired: 4 in, 1 out]
      n85 = call-poly <vilib>:"Write Key.vi"("section"=w243, "error in (no error)"=w268, "value"=w266, "key"="TEST_ENV", "refnum"=w267) -> ("error out"=w265:errorcluster, "refnum out"=w264:T17)  [unwired: 4 in, 1 out]
      n86 = call-poly <vilib>:"Write Key.vi"("section"=w243, "error in (no error)"=w265, "value"=w263, "key"="PANEL_MODE", "refnum"=w264) -> ("error out"=w259:errorcluster, "refnum out"=w260:T17)  [unwired: 4 in, 1 out]
      n87 = call-poly <vilib>:"Write Key.vi"("section"=w243, "error in (no error)"=w259, "value"=w261, "key"="CAL_MODE", "refnum"=w260) -> ("error out"=w257:errorcluster, "refnum out"=w256:T17)  [unwired: 4 in, 1 out]
      n88 = call-poly <vilib>:"Write Key.vi"("section"=w243, "error in (no error)"=w257, "value"=w254, "key"="PANEL_TYPE", "refnum"=w256) -> ("error out"=w250:errorcluster, "refnum out"=w253:T17)  [unwired: 4 in, 1 out]
      n89 = call-poly <vilib>:"Write Key.vi"("section"=w243, "error in (no error)"=w250, "value"=w251, "key"="BAND", "refnum"=w253) -> ("error out"=w247:errorcluster, "refnum out"=w249:T17)  [unwired: 4 in, 1 out]
      n90 = call-poly <vilib>:"Write Key.vi"("section"=w243, "error in (no error)"=w247, "value"=w246, "key"="TILE", "refnum"=w249) -> ("error out"=w245:errorcluster, "refnum out"=w244:T17)  [unwired: 4 in, 1 out]
      n91 = call-poly <vilib>:"Write Key.vi"("section"=w243, "error in (no error)"=w245, "value"=w241, "key"="API_DROP", "refnum"=w244) -> ("error out"=w240:errorcluster, "refnum out"=w239:T17)  [unwired: 4 in, 1 out]
    }
    frame #2 {
      # "Panel Selections: Channels Cluster\nTX1\nTX2\nTX3\nTX4\nTXx3\nTXx4\nRX1\nRX2\nRX3\nRX4\nRXx3\nRXx4\nTx\nRx"
      n92 = Cluster To Array(cluster="Channels Cluster") -> (array=w283:bool[])
      n93 = for {
        tunnel: string[] ["PANEL_TX1", "PANEL_TX2", "PANEL_TX3", "PANEL_TX4", "PANEL_TXx3", "PANEL_TXx4", "PANEL_RX1", "PANEL_RX2", "PANEL_RX3", "PANEL_RX4", "PANEL_RXx3", "PANEL_RXx4", "PANEL_TX", "PANEL_RX"] -> [w286] mode=indexing
        shift-right: [w288] -> w279
        shift-left: w282 -> [w289]
        shift-right: [w287] -> w280
        shift-left: w281 -> [w290]
        tunnel: w283 -> [w293]
        i -> [w292]
        n94 = Index Array(array=w293, index=w292) -> (element=w291:bool)
        n95 = call-poly <vilib>:"Write Key.vi"("section"="Channels_Cluster", "error in (no error)"=w290, "value"=w291, "key"=w286, "refnum"=w289) -> ("error out"=w287:errorcluster, "refnum out"=w288:T17)  [unwired: 4 in, 1 out]
      }
    }
    frame #3 {
      # "Panel Selections: Target Devices"
      n96 = flat-sequence {
        tunnel: w301 -> [w309]
        tunnel: w300 -> [w308]
        tunnel: [w306] -> w299
        tunnel: [w305] -> w298
        tunnel: [w302] -> w295
        tunnel: w299 -> [w339]
        tunnel: w298 -> [w338]
        tunnel: [w335] -> w297
        tunnel: [w334] -> w296
        tunnel: w295 -> [w333]
        frame #0 {
          n97 = Unbundle("Target Devices Cluster") -> ("Target Devices"=w303:T18, "Target String"=w302:string)
          n98 = Cluster To Array(cluster=w303) -> (array=w307:T19)
          n99 = for {
            N: 2 -> [_]
            shift-right: [w316] -> w305
            shift-left: w309 -> [w319]
            shift-right: [w315] -> w306
            shift-left: w308 -> [w317]
            tunnel: w307 -> [w314]
            i -> [w313]
            n100 = Increment(x=w313) -> (x+1=w318:i32)
            n101 = Index Array(array=w314, index=w313) -> (element=w312:T20)
            n102 = Cluster To Array(cluster=w312) -> (array=w311:bool[])
            n103 = for {
              N: 24 -> [_]
              shift-right: [w322] -> w316
              shift-left: w319 -> [w328]
              tunnel: w318 -> [w330]
              shift-right: [w321] -> w315
              shift-left: w317 -> [w329]
              tunnel: w311 -> [w325]
              i -> [w324]
              n104 = Index Array(array=w325, index=w324) -> (element=w323:bool)
              n105 = Increment(x=w324) -> (x+1=w331:i32)
              n106 = Format Into String(format string="P%u_D%u", w330, w331) -> (resulting string=w326:string)  [unwired: 2 in, 1 out]
              n107 = call-poly <vilib>:"Write Key.vi"("section"="Target_Devices", "error in (no error)"=w329, "value"=w323, "key"=w326, "refnum"=w328) -> ("error out"=w321:errorcluster, "refnum out"=w322:T17)  [unwired: 4 in, 1 out]
            }
          }
        }
        frame #1 {
          n108 = call-poly <vilib>:"Write Key.vi"("section"="Target_Devices", "error in (no error)"=w339, "value"=w333, "key"="TARGET_STRING", "refnum"=w338) -> ("error out"=w334:errorcluster, "refnum out"=w335:T17)  [unwired: 4 in, 1 out]
        }
      }
    }
    frame #4 {
      # "Panel Selections: Beam Rotation"
      n109 = Index Array(array="Beam Rotation", index (col)=0 ("disabled index (col)")) -> (element=w342:string[])  [unwired: 1 in]
      n110 = for {
        tunnel: string[] ["ROT_TX1", "ROT_TX2", "ROT_TX3", "ROT_TX4", "ROT_TXx3", "ROT_TXx4", "ROT_RX1", "ROT_RX2", "ROT_RX3", "ROT_RX4", "ROT_RXx3", "ROT_RXx4"] -> [w355] mode=indexing
        shift-right: [w349] -> w340
        shift-left: w346 -> [w353]
        shift-right: [w348] -> w341
        shift-left: w345 -> [w354]
        tunnel: w342 -> [w352]
        i -> [w351]
        n111 = Index Array(array=w352, index=w351) -> (element=w350:string)
        n112 = call-poly <vilib>:"Write Key.vi"("section"="Beam_Rotation", "error in (no error)"=w353, "value"=w350, "key"=w355, "refnum"=w354) -> ("error out"=w349:errorcluster, "refnum out"=w348:T17)  [unwired: 4 in, 1 out]
      }
    }
    frame #5 {
      w365 = "Panel_RF_Parameters"
      # "RF Parameters: Panel Selections"
      n113 = Unbundle By Name("RF Parameters Settings Cluster") -> ("Tx RF \nFrequency"=w360:dbl, "RF Bandwidth \n(MHz)"=w359:i32, "Tx VGA"=w358:i32[], "Rx VGA"=w357:i32[])
      n114 = call-poly <vilib>:"Write Key.vi"("section"=w365, "error in (no error)"=w376, "value"=w360, "key"="PANEL_TX_FREQ", "refnum"=w374) -> ("error out"=w372:errorcluster, "refnum out"=w373:T17)  [unwired: 4 in, 1 out]
      n115 = call-poly <vilib>:"Write Key.vi"("section"=w365, "error in (no error)"=w372, "value"=w359, "key"="PANEL_BW", "refnum"=w373) -> ("error out"=w370:errorcluster, "refnum out"=w369:T17)  [unwired: 4 in, 1 out]
      n116 = for {
        N: 4 -> [_]
        shift-right: [w391] -> w367
        shift-left: w369 -> [w393]
        shift-right: [w390] -> w366
        shift-left: w370 -> [w389]
        tunnel: w365 -> [w392]
        tunnel: w358 -> [w396]
        i -> [w395]
        n117 = Index Array(array=w396, index=w395) -> (element=w394:i32)
        n118 = Increment(x=w395) -> (x+1=w397:i32)
        n119 = Format Into String(format string="PANEL_VGA_TX%u", w397) -> (resulting string=w388:string)  [unwired: 2 in, 1 out]
        n120 = call-poly <vilib>:"Write Key.vi"("section"=w392, "error in (no error)"=w389, "value"=w394, "key"=w388, "refnum"=w393) -> ("error out"=w390:errorcluster, "refnum out"=w391:T17)  [unwired: 4 in, 1 out]
      }
      n121 = for {
        N: 4 -> [_]
        shift-right: [w380] -> w363
        shift-left: w367 -> [w382]
        shift-right: [w379] -> w362
        shift-left: w366 -> [w378]
        tunnel: w365 -> [w381]
        tunnel: w357 -> [w385]
        i -> [w384]
        n122 = Index Array(array=w385, index=w384) -> (element=w383:i32)
        n123 = Increment(x=w384) -> (x+1=w386:i32)
        n124 = Format Into String(format string="PANEL_VGA_RX%u", w386) -> (resulting string=w377:string)  [unwired: 2 in, 1 out]
        n125 = call-poly <vilib>:"Write Key.vi"("section"=w381, "error in (no error)"=w378, "value"=w383, "key"=w377, "refnum"=w382) -> ("error out"=w379:errorcluster, "refnum out"=w380:T17)  [unwired: 4 in, 1 out]
      }
    }
    frame #6 {
      w411 = "Action_Set_Beam"
      # "Panel Action: Set Beam"
      n126 = Unbundle By Name("Set Beam Settings Cluster") -> ("IQ Calibration"=w405:bool, "Temperature Loop"=w404:bool, "RF Calibration"=w403:bool, "Rotate Beam"=w402:bool, "Source"=w401:T21, "Destination"=w400:enum16{"CPRI", "EXT", "MEM_ADC", "MEM_DDC"}, "RxPath"=w399:enum16{"DIRECT", "MIXER"})
      n127 = call-poly <vilib>:"Write Key.vi"("section"=w411, "error in (no error)"=w428, "value"=w405, "key"="ACTION_IQ_CAL", "refnum"=w430) -> ("error out"=w425:errorcluster, "refnum out"=w427:T17)  [unwired: 4 in, 1 out]
      n128 = call-poly <vilib>:"Write Key.vi"("section"=w411, "error in (no error)"=w425, "value"=w404, "key"="ACTION_TEMP_LOOP", "refnum"=w427) -> ("error out"=w423:errorcluster, "refnum out"=w424:T17)  [unwired: 4 in, 1 out]
      n129 = call-poly <vilib>:"Write Key.vi"("section"=w411, "error in (no error)"=w423, "value"=w403, "key"="ACTION_RF_CAL", "refnum"=w424) -> ("error out"=w419:errorcluster, "refnum out"=w421:T17)  [unwired: 4 in, 1 out]
      n130 = call-poly <vilib>:"Write Key.vi"("section"=w411, "error in (no error)"=w419, "value"=w402, "key"="ACTION_ROT_BEAM", "refnum"=w421) -> ("error out"=w417:errorcluster, "refnum out"=w418:T17)  [unwired: 4 in, 1 out]
      n131 = call-poly <vilib>:"Write Key.vi"("section"=w411, "error in (no error)"=w417, "value"=w401, "key"="ACTION_SOURCE", "refnum"=w418) -> ("error out"=w414:errorcluster, "refnum out"=w415:T17)  [unwired: 4 in, 1 out]
      n132 = call-poly <vilib>:"Write Key.vi"("section"=w411, "error in (no error)"=w414, "value"=w400, "key"="ACTION_DEST", "refnum"=w415) -> ("error out"=w410:errorcluster, "refnum out"=w412:T17)  [unwired: 4 in, 1 out]
      n133 = call-poly <vilib>:"Write Key.vi"("section"=w411, "error in (no error)"=w410, "value"=w399, "key"="ACTION_RXPATH", "refnum"=w412) -> ("error out"=w408:errorcluster, "refnum out"=w407:T17)  [unwired: 4 in, 1 out]
    }
    frame #7 {
      w444 = "Action_DMA"
      # "Panel Action Settings: DMA"
      n134 = Unbundle By Name("DMA Settings Cluster") -> ("Tx Waveform File Names"=w436:string[], "State"=w435:enum16{"Start", "Stop"}, "Injection Point"=w434:enum16{"MEM_DAC", "MEM_DUC"}, "Rx File Captures"=w433:string[], "# of Samples"=w432:i32, "Capture Point"=w431:enum16{"MEM_ADC", "MEM_DDC"})
      n135 = Array Size(array=w433) -> (size(s)=w438:i32)
      n136 = Array Size(array=w436) -> (size(s)=w459:i32)
      n137 = call-poly <vilib>:"Write Key.vi"("section"=w444, "error in (no error)"=w464, "value"=w459, "key"="ACTION_DMA_TX_FILENUM", "refnum"=w463) -> ("error out"=w460:errorcluster, "refnum out"=w461:T17)  [unwired: 4 in, 1 out]
      n138 = for {
        N: w459 -> [_]
        shift-right: [w481] -> w456
        shift-left: w460 -> [w482]
        shift-right: [w483] -> w458
        shift-left: w461 -> [w484]
        tunnel: w444 -> [w480]
        tunnel: w436 -> [w478]
        i -> [w477]
        n139 = Index Array(array=w478, index=w477) -> (element=w476:string)
        n140 = Increment(x=w477) -> (x+1=w485:i32)
        n141 = Format Into String(format string="ACTION_TX_WFM_NAME%u", w485) -> (resulting string=w479:string)  [unwired: 2 in, 1 out]
        n142 = call-poly <vilib>:"Write Key.vi"("section"=w480, "error in (no error)"=w482, "value"=w476, "key"=w479, "refnum"=w484) -> ("error out"=w481:errorcluster, "refnum out"=w483:T17)  [unwired: 4 in, 1 out]
      }
      n143 = call-poly <vilib>:"Write Key.vi"("section"=w444, "error in (no error)"=w456, "value"=w435, "key"="ACTION_DMA_TX_STATE", "refnum"=w458) -> ("error out"=w454:errorcluster, "refnum out"=w453:T17)  [unwired: 4 in, 1 out]
      n144 = call-poly <vilib>:"Write Key.vi"("section"=w444, "error in (no error)"=w454, "value"=w434, "key"="ACTION_DMA_TX_INJ", "refnum"=w453) -> ("error out"=w452:errorcluster, "refnum out"=w450:T17)  [unwired: 4 in, 1 out]
      n145 = call-poly <vilib>:"Write Key.vi"("section"=w444, "error in (no error)"=w452, "value"=w438, "key"="ACTION_DMA_RX_FILENUM", "refnum"=w450) -> ("error out"=w449:errorcluster, "refnum out"=w448:T17)  [unwired: 4 in, 1 out]
      n146 = for {
        N: w438 -> [_]
        shift-right: [w470] -> w445
        shift-left: w449 -> [w471]
        shift-right: [w472] -> w446
        shift-left: w448 -> [w473]
        tunnel: w444 -> [w469]
        tunnel: w433 -> [w467]
        i -> [w466]
        n147 = Index Array(array=w467, index=w466) -> (element=w465:string)
        n148 = Increment(x=w466) -> (x+1=w474:i32)
        n149 = Format Into String(format string="ACTION_RX_WFM_NAME%u", w474) -> (resulting string=w468:string)  [unwired: 2 in, 1 out]
        n150 = call-poly <vilib>:"Write Key.vi"("section"=w469, "error in (no error)"=w471, "value"=w465, "key"=w468, "refnum"=w473) -> ("error out"=w470:errorcluster, "refnum out"=w472:T17)  [unwired: 4 in, 1 out]
      }
      n151 = call-poly <vilib>:"Write Key.vi"("section"=w444, "error in (no error)"=w445, "value"=w432, "key"="ACTION_DMA_RX_SAMPLES", "refnum"=w446) -> ("error out"=w442:errorcluster, "refnum out"=w443:T17)  [unwired: 4 in, 1 out]
      n152 = call-poly <vilib>:"Write Key.vi"("section"=w444, "error in (no error)"=w442, "value"=w431, "key"="ACTION_DMA_RX_CAPT", "refnum"=w443) -> ("error out"=w439:errorcluster, "refnum out"=w440:T17)  [unwired: 4 in, 1 out]
    }
    frame #8 {
      w499 = "Action_MBCFR"
      # "Panel Action Settings: MBCFR"
      n153 = Unbundle By Name("MB-CFR Settings Cluster") -> ("Individual\nEnable"=w493:bool, "Individual\nThreshold"=w492:dbl, "Individual\nDelta"=w491:dbl, "Individual\nWeight"=w490:dbl, "Combined\nEnable"=w489:bool, "Combined\nThreshold"=w488:dbl, "Combined\nDelta"=w487:dbl)
      n154 = call-poly <vilib>:"Write Key.vi"("section"=w499, "error in (no error)"=w518, "value"=w493, "key"="ACTION_MBCFR_IND_EN", "refnum"=w517) -> ("error out"=w514:errorcluster, "refnum out"=w515:T17)  [unwired: 4 in, 1 out]
      n155 = call-poly <vilib>:"Write Key.vi"("section"=w499, "error in (no error)"=w514, "value"=w492, "key"="ACTION_MBCFR_IND_THR", "refnum"=w515) -> ("error out"=w512:errorcluster, "refnum out"=w511:T17)  [unwired: 4 in, 1 out]
      n156 = call-poly <vilib>:"Write Key.vi"("section"=w499, "error in (no error)"=w512, "value"=w491, "key"="ACTION_MBCFR_IND_DEL", "refnum"=w511) -> ("error out"=w508:errorcluster, "refnum out"=w509:T17)  [unwired: 4 in, 1 out]
      n157 = call-poly <vilib>:"Write Key.vi"("section"=w499, "error in (no error)"=w508, "value"=w490, "key"="ACTION_MBCFR_IND_WT", "refnum"=w509) -> ("error out"=w505:errorcluster, "refnum out"=w506:T17)  [unwired: 4 in, 1 out]
      n158 = call-poly <vilib>:"Write Key.vi"("section"=w499, "error in (no error)"=w505, "value"=w489, "key"="ACTION_MBCFR_CMB_EN", "refnum"=w506) -> ("error out"=w501:errorcluster, "refnum out"=w503:T17)  [unwired: 4 in, 1 out]
      n159 = call-poly <vilib>:"Write Key.vi"("section"=w499, "error in (no error)"=w501, "value"=w488, "key"="ACTION_MBCFR_CMB_THR", "refnum"=w503) -> ("error out"=w498:errorcluster, "refnum out"=w500:T17)  [unwired: 4 in, 1 out]
      n160 = call-poly <vilib>:"Write Key.vi"("section"=w499, "error in (no error)"=w498, "value"=w487, "key"="ACTION_MBCFR_CMB_DEL", "refnum"=w500) -> ("error out"=w495:errorcluster, "refnum out"=w496:T17)  [unwired: 4 in, 1 out]
    }
    frame #9 {
      w523 = "Panel_Action_Sequence"
      # "Panel Action Sequence List"
      n161 = Array Size(array="Panel Action Sequence") -> (size(s)=w519:i32)
      n162 = call-poly <vilib>:"Write Key.vi"("section"=w523, "error in (no error)"=w527, "value"=w519, "key"="PANEL_SEQ_NUM", "refnum"=w528) -> ("error out"=w524:errorcluster, "refnum out"=w525:T17)  [unwired: 4 in, 1 out]
      n163 = for {
        N: w519 -> [_]
        shift-right: [w537] -> w521
        shift-left: w525 -> [w534]
        shift-right: [w536] -> w520
        shift-left: w524 -> [w532]
        tunnel: w523 -> [w535]
        tunnel: "Panel Action Sequence" -> [w531]
        i -> [w530]
        n164 = Increment(x=w530) -> (x+1=w538:i32)
        n165 = Index Array(array=w531, index=w530) -> (element=w529:T6)
        n166 = Format Into String(format string="PANEL_SEQ_INDEX%u", w538) -> (resulting string=w533:string)  [unwired: 2 in, 1 out]
        n167 = call-poly <vilib>:"Write Key.vi"("section"=w535, "error in (no error)"=w532, "value"=w529, "key"=w533, "refnum"=w534) -> ("error out"=w536:errorcluster, "refnum out"=w537:T17)  [unwired: 4 in, 1 out]
      }
    }
  }
  n168 = call <vilib>:"Close Config Data.vi"("error in (no error)"=w1, "refnum"=w2) -> ("error out"=→"error out":errorcluster)  [unwired: 1 in, 8 out]
